vi "SandboxNeadleValve.vi"() -> ()   [LabVIEW 2019]
uses:
  TypeDef/Needle Valve Data.ctl
  modbus engine custom/MB_ENGINE_class/Engine State.ctl
  TypeDef/Needle Valve State.ctl
  modbus engine custom/MB_ENGINE_class/Engine Alarms.ctl
  modbus engine custom/MB_ENGINE_class/Settings.ctl
  modbus engine custom/MB_ENGINE_class/Limits Status.ctl
  TypeDef/Needle Valve Settings.ctl
  FPGA/TypeDef/DO index.ctl
  Database_Postgress_class/Database_Postgress.lvclass
  C:/Users/H4001/Documents/GitHub/H4000/src/DatabaseInterface_class/DatabaseInterface.lvclass
  Database_Postgress_class/Connection Info.ctl
  Logger_class/Logger.lvclass
  ConfigJSON_class/ConfigJSON.lvclass
  C:/Users/H4001/Documents/GitHub/H4000/src/ConfigInterface_class/ConfigInterface.lvclass
  MessageAMC_class/MessageAMC.lvclass
  C:/Users/H4001/Documents/GitHub/H4000/src/MessageInterface_class/MessageInterface.lvclass
  FPGA_API_class/FPGA API.lvclass
  ConfigJSON_class/ConfigJSON.lvclass/ConfigJSON.ctl
  NeedleValve_class/NeedleValve.lvclass
  SV_Puplisher_class/SV_Publisher.lvclass
  DatabaseInterface_class/DatabaseInterface.lvclass
  MessageInterface_class/MessageInterface.lvclass
  <vilib>/NI/AMC/AMC.lvlib
  modbus engine custom/MB_ENGINE_class/MB_ENGINE.lvclass
panel:
  out "Numeric 2":i32
  out "Numeric":i32
  out "error out 3":errorcluster
  in  "value":bool=TRUE
  in  "Time uSec":u32=1000000
  in  "#DO":T1=24 items=["DO 0 [KP1 [DO 0]]", "DO 1 [ON KP2 [DO 1]]", "DO 2 [ON KP3 [DO 2]]", "DO 3 [WATER Y18.1 [DO3]]", "DO 4 [WATER Y18.2 [DO4]]", "DO 5 [KP6 Y29.1 33.7]", "DO 6 [KP7 Y29.2 33.8]", "DO 7 [KP8 Y29.3 33.9]", "DO 8 [KP9 Y29.4  33.12]", "DO 9 [KP10 Y29.5 33.1]", "DO 10 [KP11 Y29.6 33.2]", "DO 11 [KP12 Y29.7  33.13]", "DO 12 [KP13 Y29.8  33.11]", "DO 13 [KP14 Y29.9 33.10]", "DO 14 [KP15 Y29.10  33.6]", "DO 15 [KP16 Y29.11  33.5]", "DO 16 [KP17 Y29.12  33.4]", "DO 17 [KP18 Y29.13 33.3]", "DO 18 [AIR KP19]", "DO 19 [STEP DRIVE EN KP20]", "DO 20 [KP21 Y44.1 OPEN]", "DO 21 [ KP22 Y44.1 CLOSE]", "DO 22 [ KP23 Y44.2 OPEN]", "DO 23", "DO 24 [STEP DRIVE 1]", "DO 25 [STEP DRIVE 2]"]
  in  "set":bool
  out "DO":bool[](array[boolean])
  out "step":i32(graph)
  out "encoder":i32(graph)
  in  "Needle Valve Settings":T2={"average size"=100, "open force"=40, "close force"=20, "open settings"={"ACC Steps Per Sec^2"=51, "DEC Steps Per Sec^2"=51, "Min Velosity Step Per Sec"=51, "Max Velosity Step Per Sec"=101, "MicroStep"=16}, "close settings"={"ACC Steps Per Sec^2"=52, "DEC Steps Per Sec^2"=52, "Min Velosity Step Per Sec"=52, "Max Velosity Step Per Sec"=102, "MicroStep"=16}}
  out "NVM_1_DATA":T4={"Engine State"=8, "StateValveModbus"=enum."IDLE", "Alarms"={"OL"=FALSE, "TF"=FALSE, "STL"=FALSE, "OCP"=FALSE, "CPUV"=FALSE, "UVLO"=FALSE, "SPI_ERROR"=FALSE, "Fault"=FALSE, "OL 2"=FALSE, "TF 2"=FALSE, "STL 2"=FALSE, "OCP 2"=FALSE, "CPUV 2"=FALSE, "UVLO 2"=FALSE, "reserved"=TRUE, "InitDone"=TRUE}, "RAW Possition"=124110, "Angele"=0.0, "Step"=0, "Encoder"=0, "Kinematic"={"ACC Steps Per Sec^2"=100, "DEC Steps Per Sec^2"=100, "Min Velosity Step Per Sec"=100, "Max Velosity Step Per Sec"=200, "MicroStep"=16}, "Limits"={"Fault 2 Switch"=FALSE, "Fault 1 Switch"=FALSE, "Center(Home)"=FALSE, "Lower Limit"=FALSE, "Upper Limit"=FALSE}} {"Engine State" items=["ACCELERATING", "DECELERATINGTOSTOP", "DECELERATING", "STEADY", "INDEX_ACCEL", "NDEX_RUN", "INDEX_DECEL", "INDEX_DWELL", "INACTIVE", "STANDBY", "STANDBYTOINACTIVE"]}
  in  "SET_SETTINGS":bool
  in  "clear":bool
  in  "stop":bool
  in  "close":bool
  in  "open":bool
  out "UDP port used":u16
  out "error out 2":errorcluster
  out "error out":errorcluster
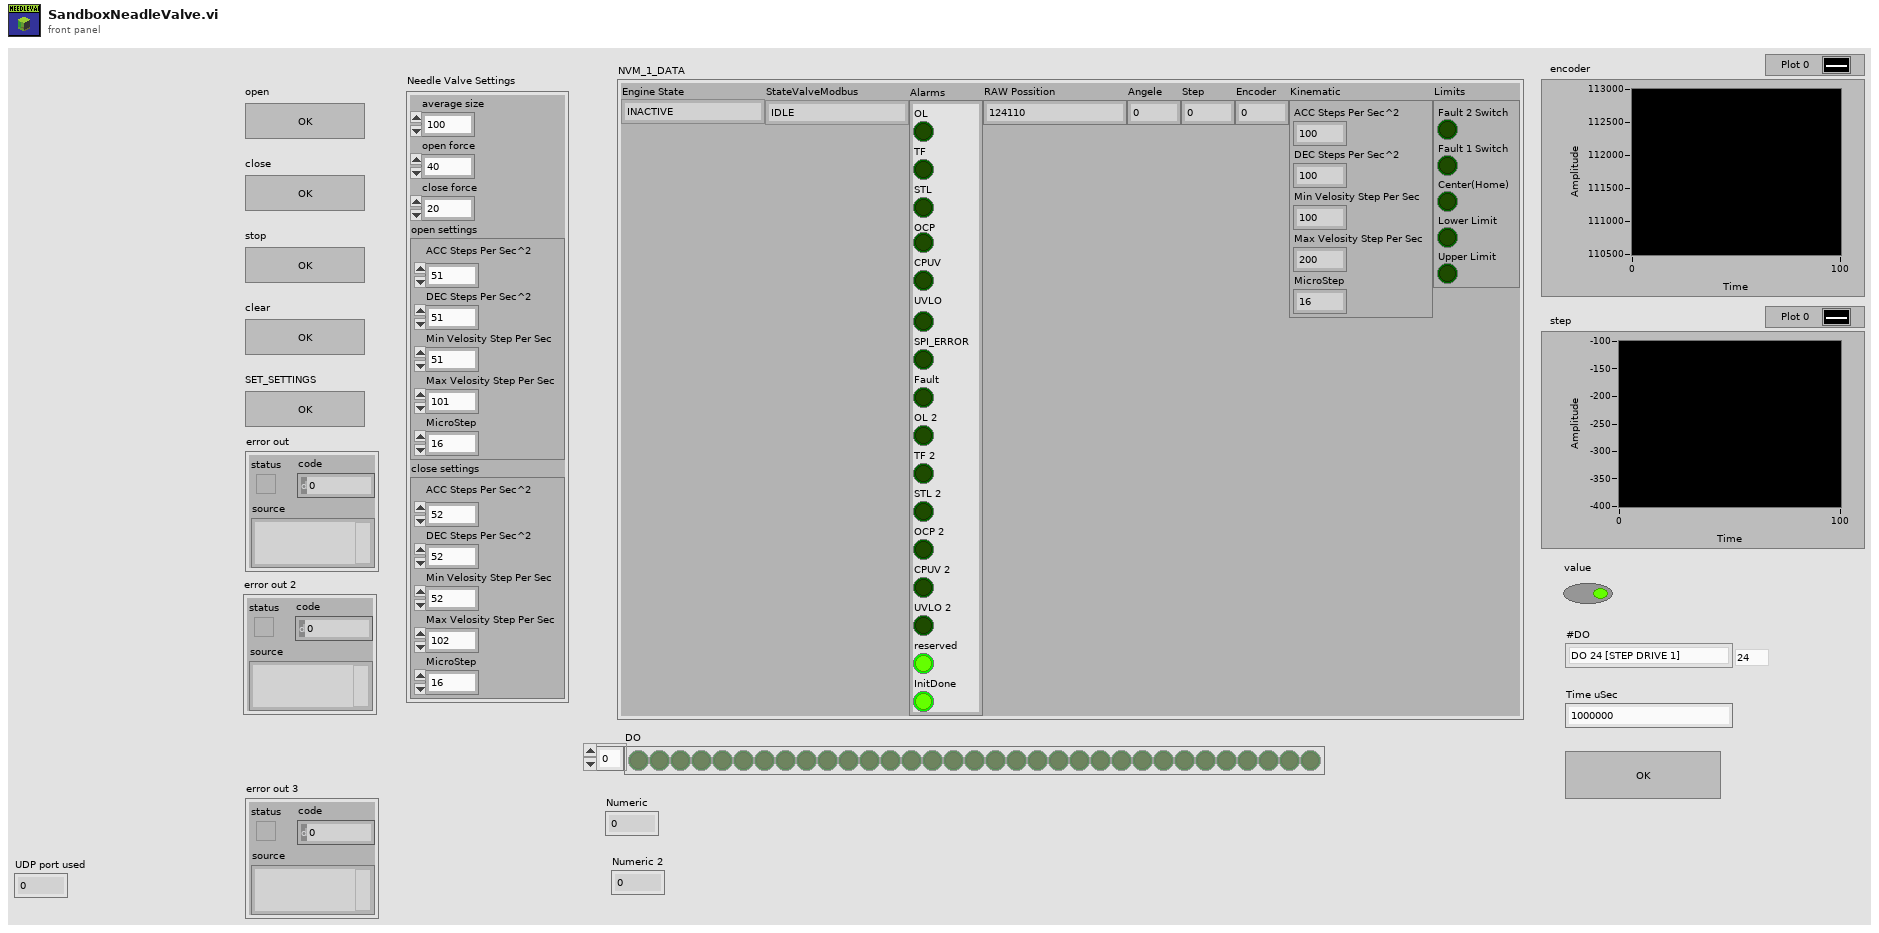
[diagram p1: front panel]
types:
  T1 = typedef "DO index.ctl" = u8
  T2 = typedef "Needle Valve Settings.ctl" = cluster{"average size":i32, "open force":u16, "close force":u16, "open settings":T3, "close settings":T3}
  T3 = typedef "MB_ENGINE.lvclass/Settings.ctl" = cluster{"ACC Steps Per Sec^2":u16, "DEC Steps Per Sec^2":u16, "Min Velosity Step Per Sec":u16, "Max Velosity Step Per Sec":u16, "MicroStep":u16}
  T4 = typedef "Needle Valve Data.ctl" = cluster{"Engine State":T5, "StateValveModbus":T6, "Alarms":T7, "RAW Possition":i32, "Angele":dbl, "Step":i32, "Encoder":i32, "Kinematic":T3, "Limits":T8}
  T5 = typedef "MB_ENGINE.lvclass/Engine State.ctl" = u16
  T6 = typedef "Needle Valve State.ctl" = enum16{"IDLE", "OPENING", "CLOSING", "STOP"}
  T7 = typedef "MB_ENGINE.lvclass/Engine Alarms.ctl" = cluster{"OL":bool, "TF":bool, "STL":bool, "OCP":bool, "CPUV":bool, "UVLO":bool, "SPI_ERROR":bool, "Fault":bool, "OL 2":bool, "TF 2":bool, "STL 2":bool, "OCP 2":bool, "CPUV 2":bool, "UVLO 2":bool, "reserved":bool, "InitDone":bool}
  T8 = typedef "MB_ENGINE.lvclass/Limits Status.ctl" = cluster{"Fault 2 Switch":bool, "Fault 1 Switch":bool, "Center(Home)":bool, "Lower Limit":bool, "Upper Limit":bool}
  T9 = typedef "DatabaseInterface.lvclass/Connection Info.ctl" = cluster{"IP_Address":string, "Port":u16, "Timeout":i32, "User":string, "Password":string, "Database":string}
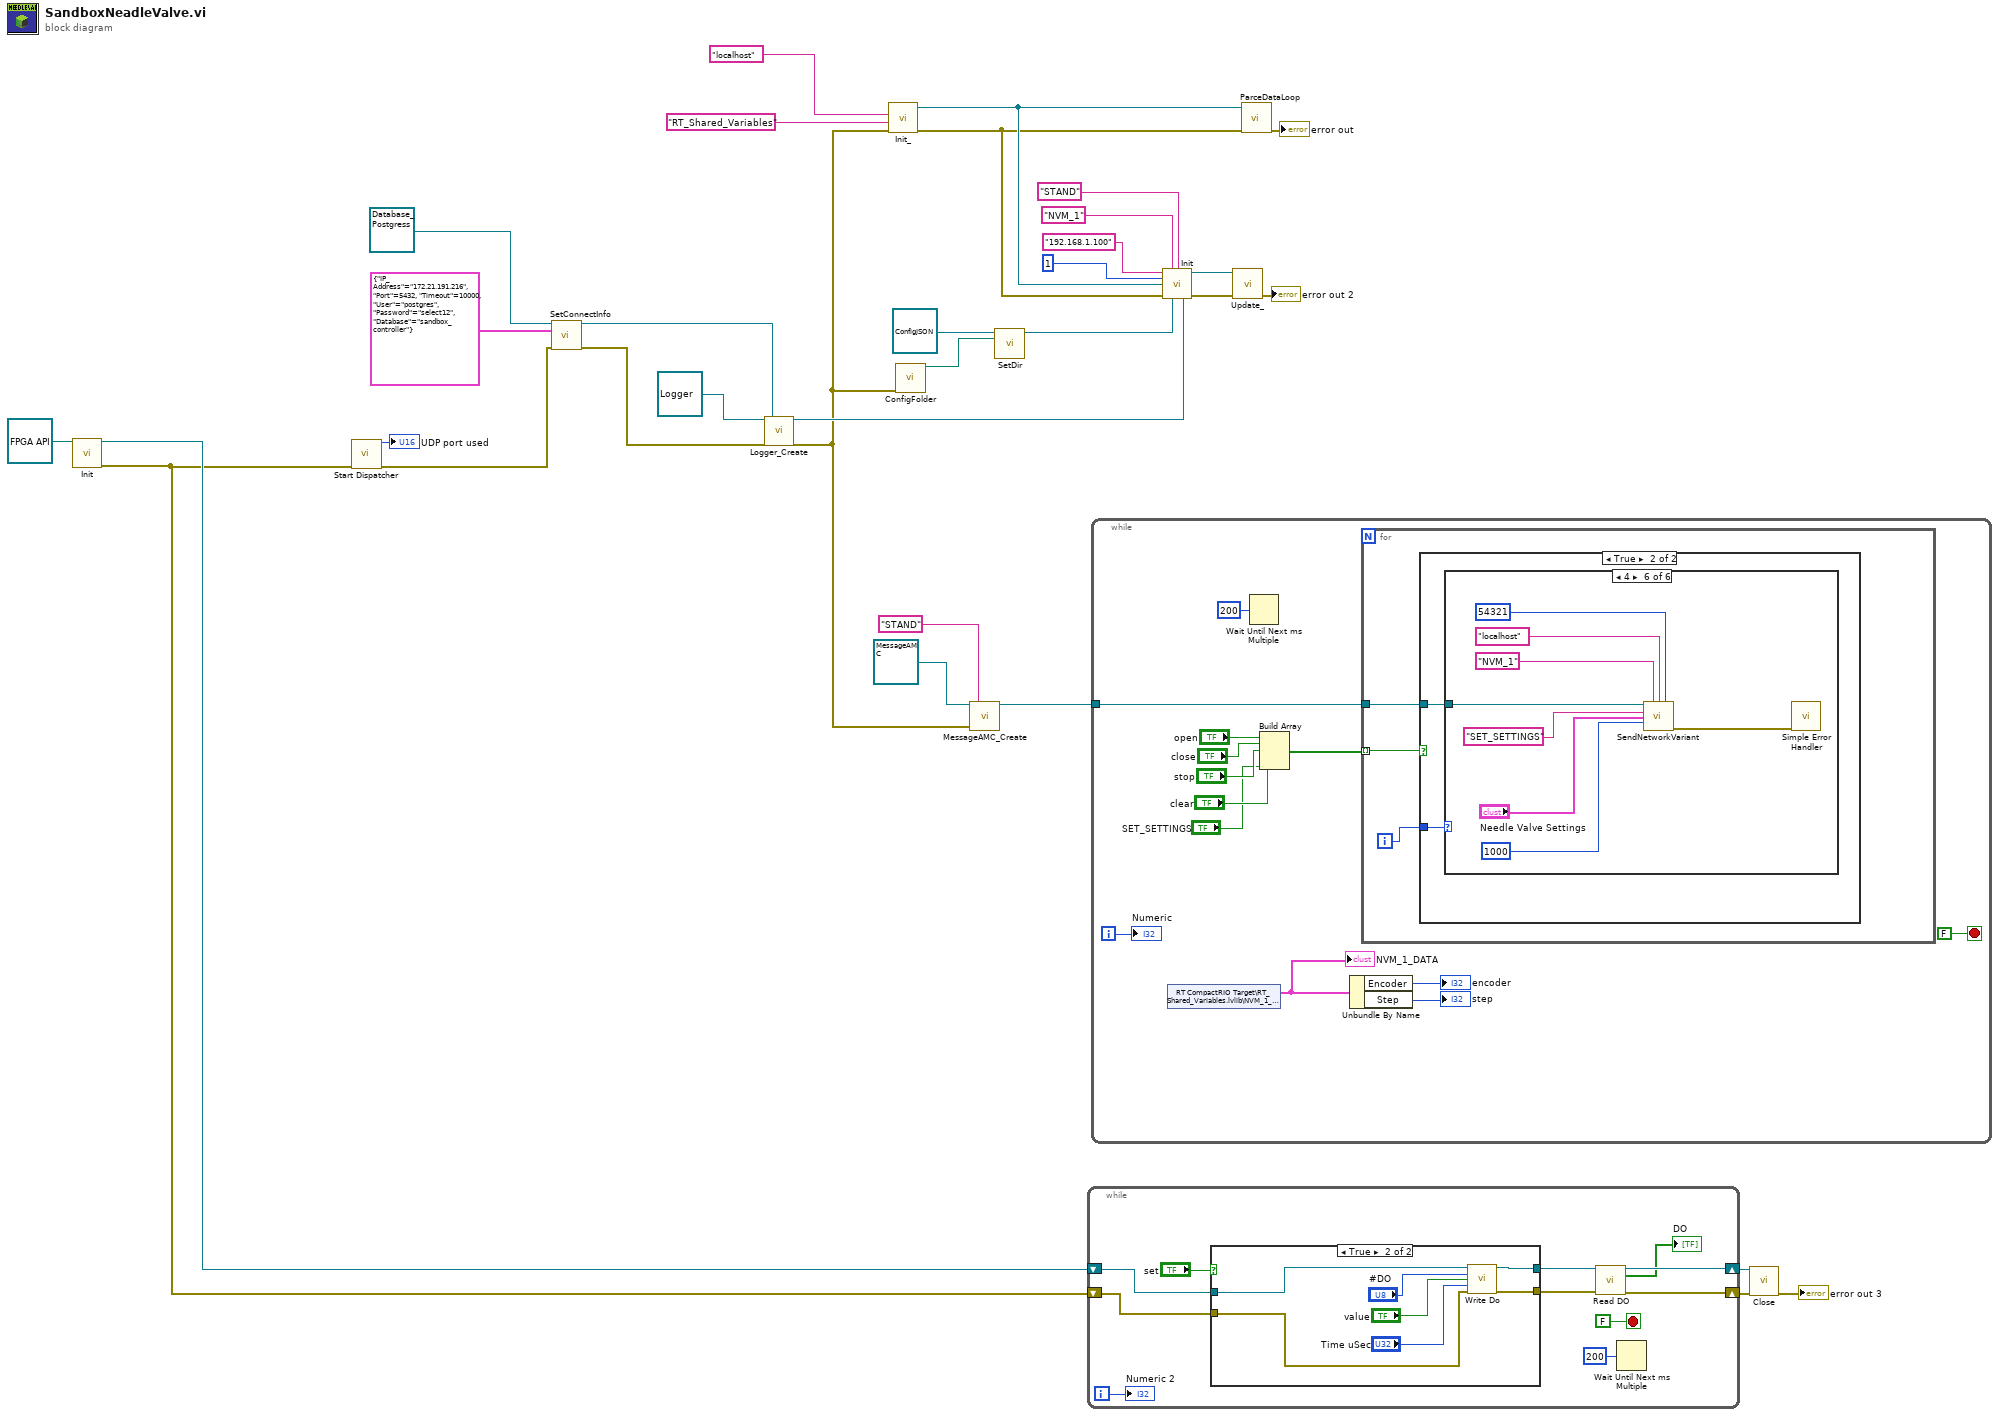
[diagram p0: block diagram]
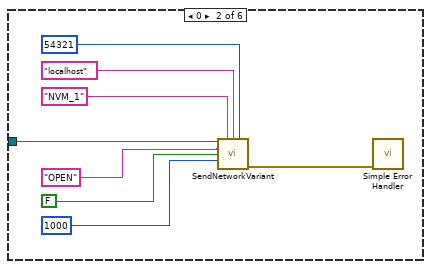
[diagram p5: hidden frame]
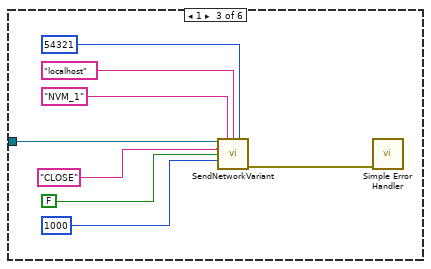
[diagram p6: hidden frame]
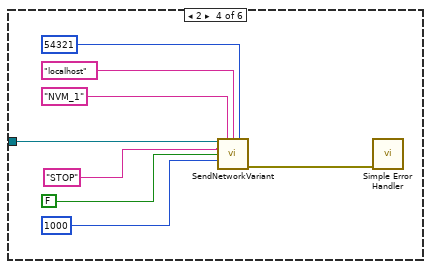
[diagram p7: hidden frame]
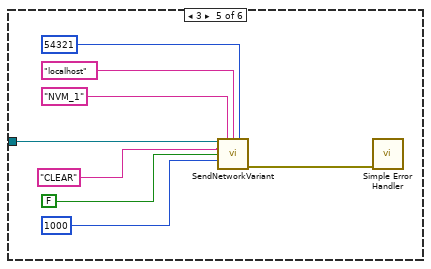
[diagram p8: hidden frame]
diagram:
  n1 = call "Init.vi"("FPGA API in"=refnum<class "FPGA API.lvclass"> refnum) -> ("FPGA API out"=w9:refnum<class "FPGA API.lvclass">, "error out"=w8:errorcluster)  [unwired: 13 in]
  n2 = call <vilib>:"Start Dispatcher.vi"("error in"=w8) -> ("UDP port used"=→"UDP port used":u16, "error out"=w15:errorcluster)  [unwired: 12 in, 1 out]
  n3 = call-dynamic "SetConnectInfo.vi"("reference in"=refnum<class "Database_Postgress.lvclass"> refnum, "Connection Info"=T9 {"IP_Address"="172.21.191.216", "Port"=5432, "Timeout"=10000, "User"="postgres", "Password"="select12", "Database"="sandbox_controller"}, "error in (no error)"=w15) -> ("reference out"=w22:refnum<class "Database_Postgress.lvclass">, "error out"=w21:errorcluster)  [unwired: 11 in]
  n4 = call "Logger_Create.vi"("reference in"=refnum<class "Logger.lvclass"> refnum, "error in (no error)"=w21, "DatabaseInterface"=w22) -> ("reference out"=w17:refnum<class "Logger.lvclass">, "error out"=w11:errorcluster)  [unwired: 15 in]
  n5 = call "Init_.vi"("error in (no error)"=w11, "lib"="RT_Shared_Variables", "host"="localhost") -> ("error out"=w26:errorcluster, "SV_Publisher out"=w27:refnum<class "SV_Publisher.lvclass">)  [unwired: 7 in]
  n6 = call "ConfigFolder.vi"("error in (no error)"=w11) -> ("dup path"=w19:path)  [unwired: 13 in, 1 out]
  n7 = call "MessageAMC_Create.vi"("reference in"=refnum<class "MessageAMC.lvclass"> refnum ("MessageAMC"), "error in (no error)"=w11, "message queue name"="STAND") -> ("amc"=w13:refnum<class "MessageAMC.lvclass">)  [unwired: 15 in, 1 out]
  n8 = call "SetDir.vi"("reference in"=refnum<class "ConfigJSON.lvclass"> refnum ("ConfigJSON"), "Config Dir"=w19) -> ("JSON"=w18:refnum<class "ConfigJSON.lvclass">)  [unwired: 13 in]
  n9 = while {
    shift-right: [w39] -> w3
    shift-left: w9 -> [w42]
    shift-right: [w37] -> w2
    shift-left: w8 -> [w41]
    i -> [w34]
    stop <- FALSE stop-if-true
    n10 = case shown="True" "set" {
      tunnel: [w46 w53] -> w40
      tunnel: [w45 w52] -> w38
      tunnel: w42 -> [w46 w48]
      tunnel: w41 -> [w45 w51]
      frame False {
      }
      frame True {
        n11 = call "Write Do.vi"("FPGA API in"=w48, "#DO"="#DO", "value"="value", "Time uSec"="Time uSec", "error in (no error)"=w51) -> ("FPGA API out"=w53:refnum<class "FPGA API.lvclass">, "error out"=w52:errorcluster)  [unwired: 9 in]
      }
    }
    n12 = call "Read DO.vi"("FPGA API in"=w40, "error in (no error)"=w38) -> ("FPGA API out"=w39:refnum<class "FPGA API.lvclass">, "Ds"=→"DO":bool[], "error out"=w37:errorcluster)  [unwired: 11 in]
    n13 = Wait Until Next ms Multiple(millisecond multiple=u32 200) -> ()  [unwired: 1 out]
    "Numeric 2" <- w34
  }
  n14 = while {
    tunnel: w13 -> [w66]
    i -> [w54]
    stop <- FALSE stop-if-true
    n15 = shared-variable "RT CompactRIO Target\\RT_Shared_Variables.lvlib\\NVM_1_DATA"() -> (w57:T4)  [unwired: 1 in, 1 out]
    "NVM_1_DATA" <- w57
    n16 = Wait Until Next ms Multiple(millisecond multiple=u32 200 ("milliseconds to wait")) -> ()  [unwired: 1 out]
    n17 = Build Array("open", "close", "stop", "clear", "SET_SETTINGS") -> (w60:bool[])
    n18 = Unbundle By Name(w57) -> ("Encoder"=→"encoder":i32, "Step"=→"step":i32)
    n19 = for {
      tunnel: w66 -> [w69]
      tunnel: w60 -> [w68] mode=indexing
      i -> [w67]
      n20 = case shown="True" w68 {
        tunnel: w69 -> [_ w71]
        tunnel: w67 -> [_ w70]
        frame False {
        }
        frame True {
          n21 = case shown="4" w70 {
            tunnel: w71 -> [_ w73 w81 w89 w97 w106]
            frame Default {
            }
            frame 0 {
              n22 = call "SendNetworkVariant.vi"("reference in"=w73, "receiver process"="NVM_1", "receiver host"="localhost", "receiver port (0)"=u16 54321, "name"="OPEN", "data"=FALSE, "timeout (25000 ms)"=1000) -> ("error out"=w77:errorcluster)  [unwired: 6 in, 2 out]
              n23 = call <vilib>:"Simple Error Handler.vi"("error in (no error)"=w77) -> ()  [unwired: 4 in, 5 out]
            }
            frame 1 {
              n24 = call "SendNetworkVariant.vi"("reference in"=w81, "receiver process"="NVM_1", "receiver host"="localhost", "receiver port (0)"=u16 54321, "name"="CLOSE", "data"=FALSE, "timeout (25000 ms)"=1000) -> ("error out"=w85:errorcluster)  [unwired: 6 in, 2 out]
              n25 = call <vilib>:"Simple Error Handler.vi"("error in (no error)"=w85) -> ()  [unwired: 4 in, 5 out]
            }
            frame 2 {
              n26 = call "SendNetworkVariant.vi"("reference in"=w89, "receiver process"="NVM_1", "receiver host"="localhost", "receiver port (0)"=u16 54321, "name"="STOP", "data"=FALSE, "timeout (25000 ms)"=1000) -> ("error out"=w93:errorcluster)  [unwired: 6 in, 2 out]
              n27 = call <vilib>:"Simple Error Handler.vi"("error in (no error)"=w93) -> ()  [unwired: 4 in, 5 out]
            }
            frame 3 {
              n28 = call "SendNetworkVariant.vi"("reference in"=w97, "receiver process"="NVM_1", "receiver host"="localhost", "receiver port (0)"=u16 54321, "name"="CLEAR", "data"=FALSE, "timeout (25000 ms)"=1000) -> ("error out"=w101:errorcluster)  [unwired: 6 in, 2 out]
              n29 = call <vilib>:"Simple Error Handler.vi"("error in (no error)"=w101) -> ()  [unwired: 4 in, 5 out]
            }
            frame 4 {
              n30 = call "SendNetworkVariant.vi"("reference in"=w106, "receiver process"="NVM_1", "receiver host"="localhost", "receiver port (0)"=u16 54321, "name"="SET_SETTINGS", "data"="Needle Valve Settings", "timeout (25000 ms)"=1000) -> ("error out"=w109:errorcluster)  [unwired: 6 in, 2 out]
              n31 = call <vilib>:"Simple Error Handler.vi"("error in (no error)"=w109) -> ()  [unwired: 4 in, 5 out]
            }
          }
        }
      }
    }
    "Numeric" <- w54
  }
  n32 = call "Init.vi"("address"="192.168.1.100", "Name"="NVM_1", "ParentName"="STAND", "addres"=u16 1, "SV_Publisher"=w27, "error in (no error)"=w26, "ConfigInterface"=w18, "Logger"=w17) -> ("NeedleValve out"=w6:refnum<class "NeedleValve.lvclass">, "error out"=w5:errorcluster)  [unwired: 6 in]
  n33 = call "Update_.vi"("Pump_1AI_1DO_2DI in"=w6, "error in (no error)"=w5) -> ("error out"=→"error out 2":errorcluster)  [unwired: 12 in, 1 out]
  n34 = call "ParceDataLoop.vi"("error in (no error)"=w26, "SV_Publisher in"=w27) -> ("error out"=→"error out":errorcluster)  [unwired: 9 in]
  n35 = call "Close.vi"("FPGA API in"=w3, "error in (no error)"=w2) -> ("error out"=→"error out 3":errorcluster)  [unwired: 12 in, 1 out]
